vi "ADI_IMU_ADIS16470_ScaleData.vi"(4 "Received Data":u8[](array[numeric])) -> (1 "Data Array":dbl[](array[numeric]), 2 "Data Good?":bool)   [LabVIEW 2017, in "ADIS16470_IMU.lvlib"]
uses:
  ADIS16470_IMU.lvlib
panel:
  out "error out":errorcluster
  in  "error in (no error)":errorcluster
  out "Received Checksum":u16
  out "Calculated Checksum":u16
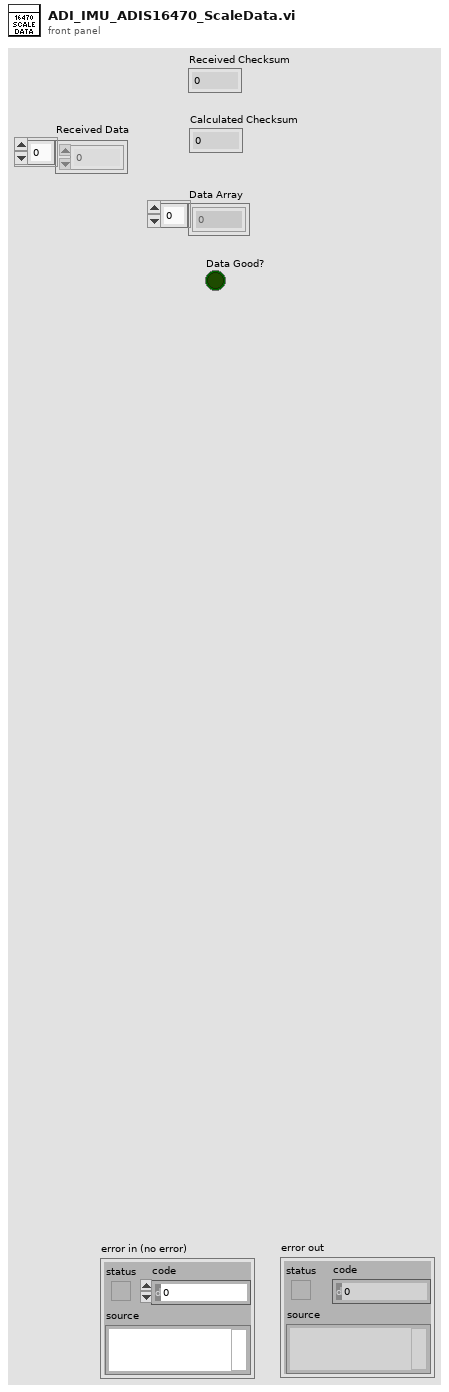
[diagram p1: front panel]
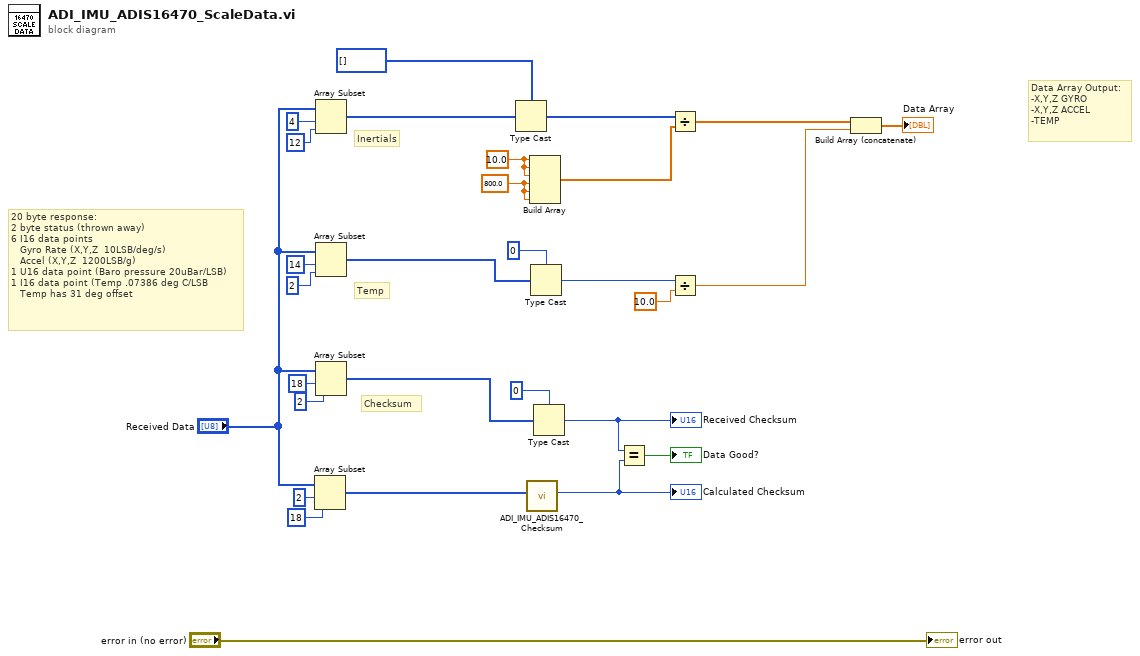
[diagram p0: block diagram]
diagram:
  w28 = 800.0
  w29 = 10.0 ("element")
  # "Checksum"
  # "Temp"
  # "Inertials"
  # "Data Array Output:\n-X,Y,Z GYRO\n-X,Y,Z ACCEL\n-TEMP"
  # "20 byte response:\n2 byte status (thrown away)\n6 I16 data points\n   Gyro Rate (X,Y,Z  10LSB/deg/s)\n   Accel (X,Y,Z  1200LSB/g)\n1 U16 data point (Baro pressure 20uBar/LSB)\n1 I16 data point (Temp .07386 deg C/LSB\n   Temp has 31 deg offset"
  n1 = Array Subset(array="Received Data", index=2, length=18) -> (w5:u8[])
  n2 = Array Subset(array="Received Data", index=4, length=12) -> (w16:u8[])
  n3 = Array Subset(array="Received Data", index=14, length=2) -> (w19:u8[])
  n4 = Array Subset(array="Received Data", index=18, length=2) -> (w10:u8[])
  n5 = Type Cast(type=i16[] [], x=w16) -> (*(type *) &x=w15:i16[])
  n6 = call "ADI_IMU_ADIS16470_Checksum.vi"("Byte Array (MSB-First)"=w5) -> ("Checksum"=w3:u16)  [unwired: 10 in]
  "Calculated Checksum" <- w3
  n7 = Build Array(w29, w29, w29, w28, w28, w28) -> (w27:dbl[])
  n8 = Type Cast(type=i16 0, x=w19) -> (*(type *) &x=w17:i16)
  n9 = Type Cast(type=u16 0, x=w10) -> (*(type *) &x=w4:u16)
  "Received Checksum" <- w4
  n10 = Equal?(x=w4, y=w3) -> (x = y?=→"Data Good?":bool)
  n11 = Divide(x=w15, y=w27) -> (x/y=w25:dbl[])
  n12 = Divide(x=w17, y=10.0 ("element")) -> (x/y=w1:dbl)
  n13 = Build Array (concatenate)(w25, w1) -> (→"Data Array":dbl[])
  "error out" <- "error in (no error)"
